vi "Test_PublicationLocked_PublisherNotOwner_Reject.vi"(8 "error in (no error)":errorcluster, 11 "TestMediator In":refnum<class "TestMediator.lvclass">) -> (0 "error out":errorcluster, 3 "TestMediator Out":refnum<class "TestMediator.lvclass">)   [LabVIEW 2017, in "TestMediator.lvclass"]
uses:
  TestMediator.lvclass
  Source/Framework/Mediator/Mediator/Mediator.lvclass
  C:/Program Files (x86)/National Instruments/LabVIEW 2017/vi.lib/ActorFramework/Actor/Actor.lvclass
  Source/Framework/IMediator/PublishRequest/PublishRequest.lvclass/PublishRequest.ctl
  Source/Framework/Transport/QueueTransport/QueueTransport.lvclass/QueueTransport.ctl
  Source/Framework/SubscriptionPolicy/BasicSubscription/BasicSubscription.lvclass/BasicSubscription.ctl
  Source/Framework/IMediator/SubscriptionRequest/SubscriptionRequest.lvclass/SubscriptionRequest.ctl
  Source/Framework/IMediator/IMediator Messages/Lock Publication Msg/Lock Publication Msg.lvclass/Lock Publication Msg.ctl
  <vilib>/ActorFramework/Message Enqueuer/Message Enqueuer.lvclass/Message Enqueuer.ctl
  Source/Framework/IMediator/IMediator Messages/Publish Msg/Publish Msg.lvclass/Publish Msg.ctl
  Source/Framework/IMediator/IMediator Messages/Subscribe Msg/Subscribe Msg.lvclass/Subscribe Msg.ctl
  <vilib>/ActorFramework/Message Enqueuer/Enqueue.vi
  Source/Framework/SubscriptionPolicy/BasicSubscription/BasicSubscription.lvclass
  C:/Git/mva-framework/Framework/IMediator/ISubscriptionPolicy/ISubscriptionPolicy.lvclass
  Source/Framework/Transport/QueueTransport/QueueTransport.lvclass
  C:/Git/mva-framework/Framework/IMediator/ITransport/ITransport.lvclass
  Source/Framework/IMediator/IMediator Messages/Lock Publication Msg/Lock Publication Msg.lvclass
  C:/Program Files (x86)/National Instruments/LabVIEW 2017/vi.lib/ActorFramework/Message/Message.lvclass
  Source/Framework/IMediator/IMediator Messages/Publish Msg/Publish Msg.lvclass
  Source/Framework/IMediator/IMediator Messages/Subscribe Msg/Subscribe Msg.lvclass
  <vilib>/ActorFramework/Stop Msg/Stop Msg.lvclass
  <vilib>/Utility/error.llb/Error Cluster From Error Code.vi
  <vilib>/ActorFramework/Message Priority Queue/Priority Enqueue.vi
  Source/Framework/IMediator/SubscriptionRequest/SubscriptionRequest.lvclass
  Source/Framework/IMediator/IPublicationPolicy/IPublicationPolicy.lvclass
  Source/Framework/IMediator/ITransport/ITransport.lvclass
  Source/Framework/IMediator/PublishRequest/PublishRequest.lvclass
  <vilib>/addons/_JKI Toolkits/VI Tester/TestCase.llb/TestCase.lvclass
  <vilib>/ActorFramework/Actor/Actor.lvclass
  Source/Framework/IMediator/ISubscriptionPolicy/ISubscriptionPolicy.lvclass
  C:/Program Files (x86)/National Instruments/LabVIEW 2017/vi.lib/addons/_JKI Toolkits/VI Tester/TestCase.llb/TestCase.lvclass
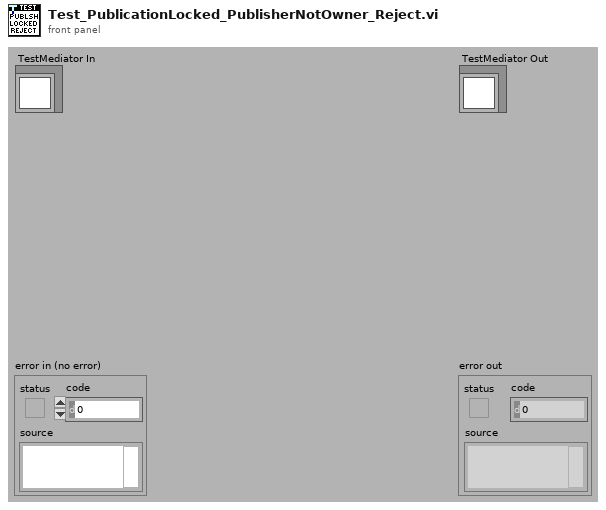
[diagram p1: front panel]
types:
  T1 = typedef "IMediator.lvlib/ISubscriptionPolicy.lvclass/ISubscriptionPolicy Reference.ctl" = refnum<data-value>
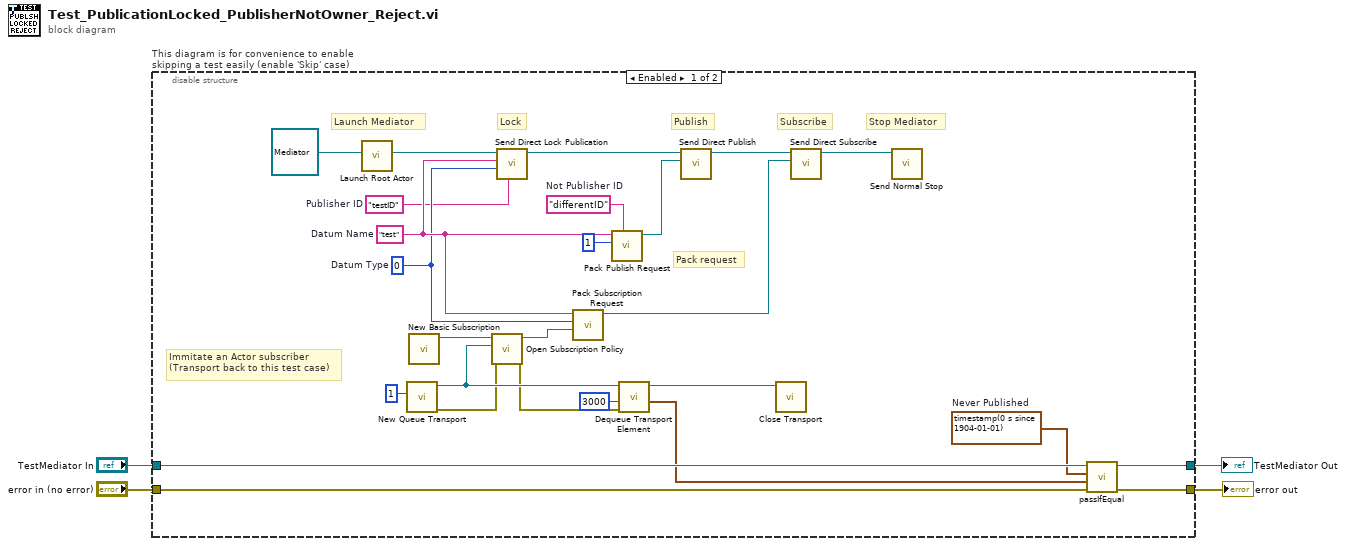
[diagram p0: block diagram]
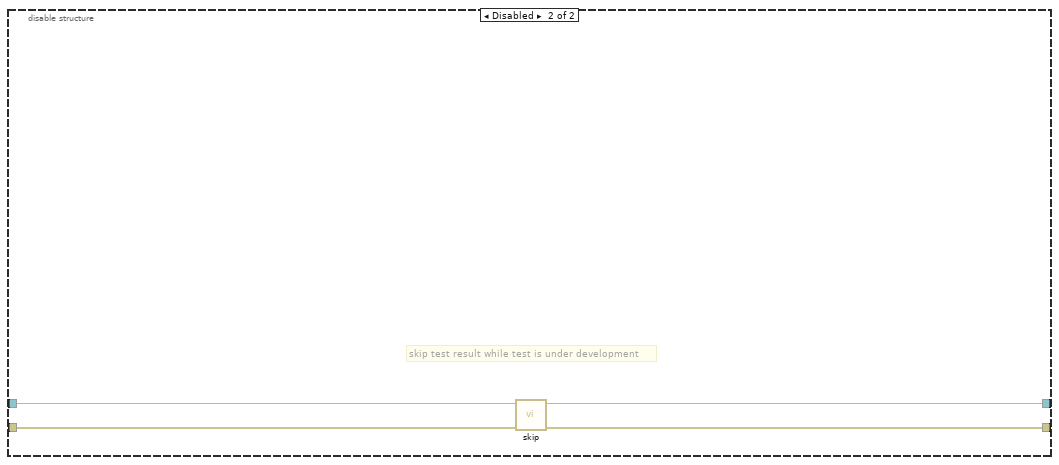
[diagram p2: hidden frame]
diagram:
  n1 = disable-structure "This diagram is for convenience to enable skipping a test easily (enable 'Skip' case)" shown="Enabled" {
    disable-tunnel: "TestMediator In" -> [w30 w34]
    disable-tunnel: [w29 w32] -> w1
    disable-tunnel: [w28 w33] -> w3
    disable-tunnel: "error in (no error)" -> [w27 w31]
    frame Enabled {
      w5 = timestamp(0 s since 1904-01-01)  # Never Published
      w7 = "differentID"  # Not Publisher ID
      w8 = "testID"  # Publisher ID
      w9 = 0  # Datum Type
      w10 = "test"  # Datum Name
      # "Immitate an Actor subscriber\n(Transport back to this test case)"
      # "Pack request"
      # "Lock"
      # "Launch Mediator"
      # "Stop Mediator"
      # "Subscribe"
      # "Publish"
      n2 = call <vilib>:"Launch Root Actor.vi"("Actor"=refnum<class "Mediator.lvclass"> refnum ("Mediator.lvlib:Mediator.lvclass")) -> ("Actor's Enqueuer"=w25:refnum<class "Message Enqueuer.lvclass">)  [unwired: 9 in, 1 out]
      n3 = call "New Queue Transport.vi"("Max Queue Size (-1)"=1) -> ("error out"=w19:errorcluster, "QueueTransport"=w21:refnum<class "QueueTransport.lvclass">)  [unwired: 9 in]
      n4 = call "New Basic Subscription.vi"() -> ("BasicSubscription Out"=w15:refnum<class "BasicSubscription.lvclass">)  [unwired: 11 in]
      n5 = call "Open Subscription Policy.vi"("error in (no error)"=w19, "Transport"=w21, "SubscriptionPolicy"=w15) -> ("error out"=w18:errorcluster, "Subscription Policy"=w14:T1)  [unwired: 7 in]
      n6 = call "Send Direct Lock Publication.vi"("Publisher ID"=w8, "Datum Type"=w9, "Datum Name"=w10, "Mediator Enqeuer"=w25) -> ("Mediator Enqueuer out"=w11:refnum<class "Message Enqueuer.lvclass">)  [unwired: 6 in, 1 out]
      n7 = call "Pack Subscription Request.vi"("Subscription Policy"=w14, "Type"=w9, "Datum Name"=w10) -> ("SubscriptionRequest"=w24:refnum<class "SubscriptionRequest.lvclass">)  [unwired: 8 in]
      n8 = call "Pack Publish Request.vi"("Publisher ID"=w7, "Data to Publish"=1, "Datum Name"=w10) -> ("PublishRequest"=w12:refnum<class "PublishRequest.lvclass">)  [unwired: 8 in]
      n9 = call "Dequeue Transport Element.vi"("error in (no error)"=w18, "Timeout In ms (-1)"=3000, "QueueTransport in"=w21) -> ("Publication Time"=w6:timestamp, "QueueTransport out"=w16:refnum<class "QueueTransport.lvclass">)  [unwired: 5 in, 2 out]
      n10 = call "Send Direct Publish.vi"("PublishRequest"=w12, "Mediator Enqeuer"=w11) -> ("Mediator Enqueuer out"=w23:refnum<class "Message Enqueuer.lvclass">)  [unwired: 8 in, 1 out]
      n11 = call-dynamic "Close Transport.vi"("QueueTransport in"=w16) -> ()  [unwired: 10 in, 1 out]
      n12 = call "Send Direct Subscribe.vi"("Subscription Request"=w24, "Message Enqueuer"=w23) -> ("Message Enqueuer out"=w17:refnum<class "Message Enqueuer.lvclass">)  [unwired: 8 in, 1 out]
      n13 = call <vilib>:"Send Normal Stop.vi"("Message Enqueuer"=w17) -> ()  [unwired: 10 in, 1 out]
      n14 = call-dynamic "passIfEqual.vi"("error in (no error)"=w27, "y"=w6, "x"=w5, "TestCase in"=w30) -> ("error out"=w28:errorcluster, "TestCase out"=w29:refnum<class "TestMediator.lvclass">)  [unwired: 6 in]
    }
    frame Disabled {
      # "skip test result while test is under development"
      n15 = call <vilib>:"skip.vi"("error in (no error)"=w31, "TestCase in"=w34) -> ("error out"=w33:errorcluster, "TestCase out"=w32:refnum<class "TestMediator.lvclass">)  [unwired: 8 in]
    }
  }
  "error out" <- w3
  "TestMediator Out" <- w1
